vi "FlexDDS-NG_DCP_Update.vi"(6 "ONLY IO_UPDATE":bool, 8 "DRCTL(true=+, false=-)":bool=TRUE, 9 "IO_UPDATE(true=u, false = '')":bool=TRUE, 10 "Channels":T1(ring), 11 "appended instruction string in":string) -> (3 "appended instruction string out":string)   [LabVIEW 2016]
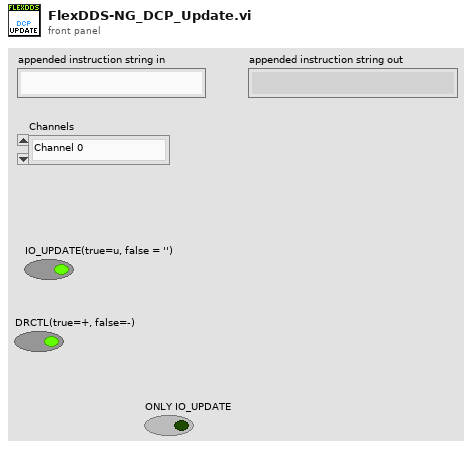
[diagram p1: front panel]
types:
  T1 = enum32{"Channel 0", "Channel 1", "Both channels"}
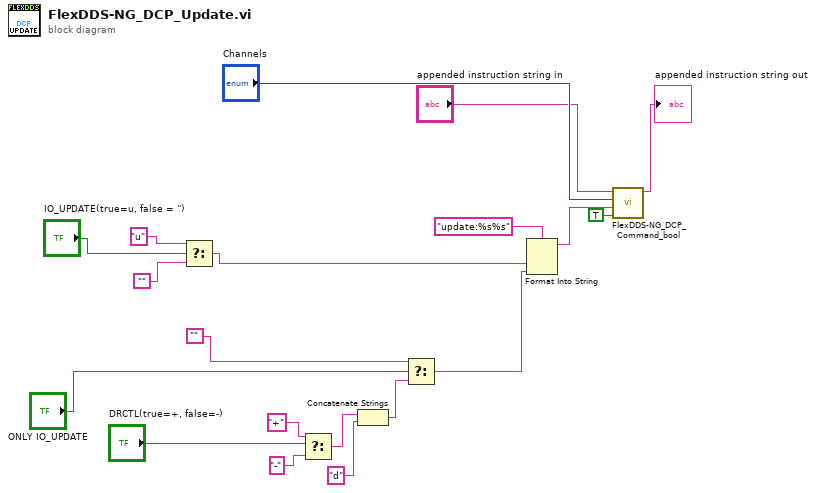
[diagram p0: block diagram]
diagram:
  n1 = Select(t="u", s="IO_UPDATE(true=u, false = '')", f="") -> (s? t:f=w2:string)
  n2 = Select(t="+", s="DRCTL(true=+, false=-)", f="-") -> (s? t:f=w5:string)
  n3 = Concatenate Strings(w5, "d" ("string")) -> (w4:string)
  n4 = Select(t="", s="ONLY IO_UPDATE", f=w4) -> (s? t:f=w1:string)
  n5 = Format Into String(format string="update:%s%s", w2, w1) -> (resulting string=w19:string)  [unwired: 2 in, 1 out]
  n6 = call "FlexDDS-NG_DCP_Command_bool.vi"("Write DCP command?"=TRUE, "command string"=w19, "Channels"="Channels", "initial instruction string"="appended instruction string in") -> ("appended instruction string"=→"appended instruction string out":string)  [unwired: 7 in]
